vi "Create Waveforms.vi"() -> (2 "core temperature":dbl[](array[numeric]), 3 "core pressure":dbl[](array[numeric]))   [LabVIEW 2018]
doc: "This is a subVI used to create simulated data for the Database Tools examples named Logging Example, Logging Example (parameterized), and Parameterized. Two arrays of simulated core pressure and core temperature data are returned."
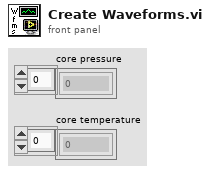
[diagram p1: front panel]
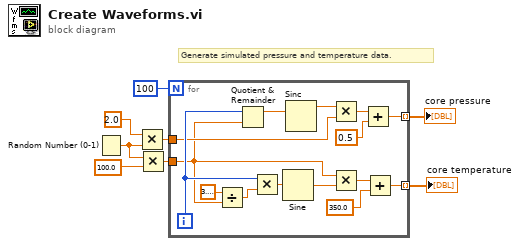
[diagram p0: block diagram]
diagram:
  # "Generate simulated pressure and temperature data."
  n1 = Random Number (0-1)() -> (number: 0 to 1=w7:dbl)
  n2 = Multiply(x=2.0, y=w7) -> (x*y=w8:dbl)
  n3 = Multiply(x=w7, y=100.0) -> (x*y=w4:dbl)
  n4 = for {
    N: 100 ("# of samples") -> [_]
    tunnel: w8 -> [w16]
    tunnel: [w19] -> w5 mode=indexing
    tunnel: [w11] -> w6 mode=indexing
    tunnel: w4 -> [w13]
    i -> [w20]
    n5 = Divide(x=3.141592653589793, y=w13) -> (x/y=w15:dbl)
    n6 = Quotient & Remainder(x=w20, y=w13) -> (x-y*floor(x/y)=w22:dbl)  [unwired: 1 out]
    n7 = Multiply(x=w20, y=w15) -> (x*y=w21:dbl)
    n8 = Sine(x=w21) -> (sin(x)=w17:dbl)
    n9 = Sinc(1:w22) -> (0:w23:dbl)
    n10 = Multiply(x=w23, y=w16) -> (x*y=w12:dbl)
    n11 = Multiply(x=w13, y=w17) -> (x*y=w18:dbl)
    n12 = Add(x=w12, y=0.5) -> (x+y=w11:dbl)
    n13 = Add(x=w18, y=350.0) -> (x+y=w19:dbl)
  }
  "core temperature" <- w5
  "core pressure" <- w6
